vi "EQ report viewer button_op.vi"   [LabVIEW 2015, in "VIPM2.lvlib"]
doc: "<b>VIP Module app: EQ report viewer</b> button.\nPregunta si obrir un report o un viewer blanc.\nGestiona per missatges si no hi ha Equalitzacions fetes.\nAlgoritme:\n - Llista equalitzacions fetes a escollir (Choose EQ to load)\n - Reconstrueix variables (EQ read summary file)\n - Mostra el resum de Layers i pixels bons, a escollir (EQ choose report)\n - Obre el EQ report viewer de la Layer (EQ report viewer x4)"
uses:
  VIPM2.lvlib
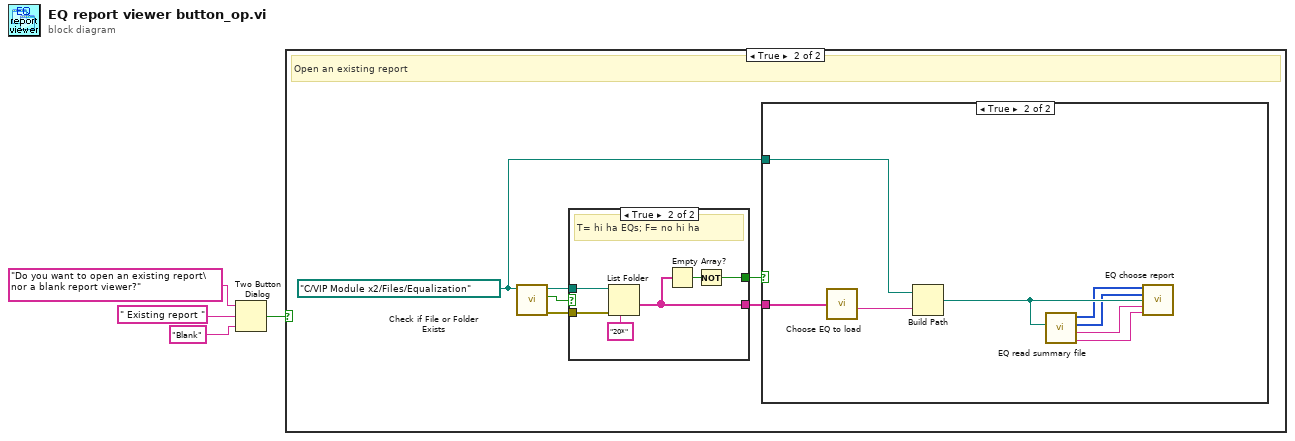
[diagram p0: block diagram]
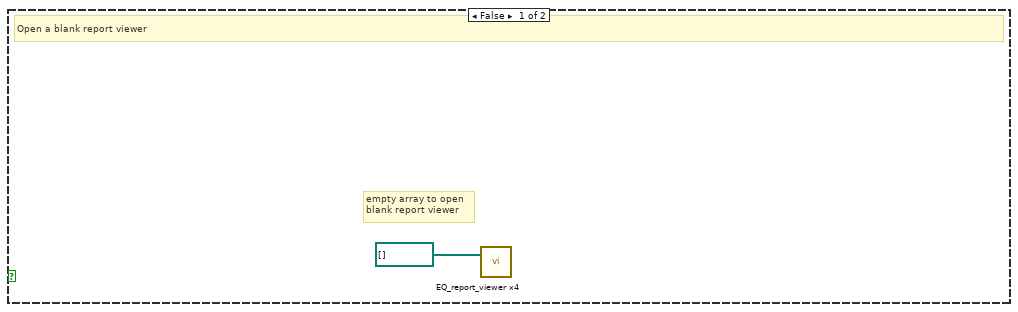
[diagram p2: hidden frame]
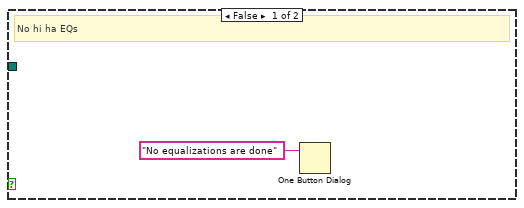
[diagram p3: hidden frame]
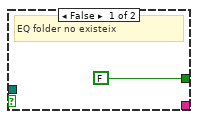
[diagram p4: hidden frame]
diagram:
  n1 = Two Button Dialog(message="Do you want to open an existing report\nor a blank report viewer?", 1:"Blank" ("F button name (\"Cancel\")"), 2:" Existing report " ("T button name (\"OK\")")) -> (T button?=w1:bool)
  n2 = case shown="True" w1 {
    frame False {
      # "empty array to open\nblank report viewer"
      # "Open a blank report viewer"
      n3 = call "EQ_report_viewer x4.vi"("folder path"=path[] []) -> ()  [unwired: 2 in]
    }
    frame True {
      w6 = path "C:/VIP Module x2/Files/Equalization" ("path")
      # "Open an existing report"
      n4 = call <vilib>:"Check if File or Folder Exists.vi"("path"=w6) -> ("error out"=w10:errorcluster, "file or folder exists?"=w11:bool, "dup path"=w9:path)  [unwired: 8 in]
      n5 = case shown="True" w11 {
        tunnel: [FALSE w22] -> w8
        tunnel: w9 -> [_ w27]
        tunnel: [_ w24] -> w7
        tunnel: w10 -> [_ w25]
        frame False {
          # "EQ folder no existeix"
        }
        frame True {
          # "T= hi ha EQs; F= no hi ha"
          n6 = List Folder(path=w27, pattern="20*", error in=w25) -> (folder names=w24:string[])  [unwired: 1 in, 3 out]
          n7 = Empty Array?(array=w24) -> (empty?=w23:bool)
          n8 = Not(x=w23) -> (.not. x?=w22:bool)
        }
      }
      n9 = case shown="True" w8 {
        tunnel: w7 -> [_ w20]
        tunnel: w6 -> [_ w18]
        frame False {
          # "No hi ha EQs"
          n10 = One Button Dialog(message="No equalizations are done") -> ()  [unwired: 1 in, 1 out]
        }
        frame True {
          n11 = call "Choose EQ to load.vi"("EQ folders"=w20) -> ("loaded EQ folder"=w19:string)  [unwired: 5 in, 2 out]
          n12 = Build Path(base path=w18, name or relative path=w19) -> (appended path=w17:path)
          n13 = call "EQ read summary file.vi"("Folder path: equalization reports"=w17) -> ("EQ summary"=w13:string, "ID summary"=w14:string, "quants px bons per chip"=w15:u8[], "ChipID list"=w16:u32[])  [unwired: 7 in]
          n14 = call "EQ choose report.vi"("Chip ID list"=w16, "quants pixels bons per Chip"=w15, "Folder path: EQ reports"=w17, "summary IDs"=w14, "summary EQ"=w13) -> ()  [unwired: 11 in]
        }
      }
    }
  }
